vi "rqp_Msg_ToServer_6.vi"(4 "Show in Debugger?":bool=TRUE, 6 "Message Priority":T1=enum."Normal", 7 "Caller in":refnum<class "Worker.lvclass">, 8 "error in":errorcluster, 10 "Data in":T2, 11 "gRPC Client in":refnum<class "gRPC Client.lvclass">) -> (0 "error out":errorcluster, 3 "dup gRPC Client out":refnum<class "gRPC Client.lvclass">, 5 "dup Caller out":refnum<class "Worker.lvclass">)   [LabVIEW 2019, in "gRPC Client (template.proto).lvlib" / "gRPC Client.lvclass"]
doc: "This VI sends a <b>Public API Request</b> message to an MHL case of the Worker that owns this VI.\n---\nThis Request matches a gRPC message of the same name."
uses:
  gRPC Client.lvclass
  C:/Program Files (x86)/National Instruments/LabVIEW 2019/vi.lib/addons/_Workers/Library/Classes/Worker/Worker.lvclass
  <vilib>/addons/_Workers/Library/Classes/Worker/Worker.lvclass
  rqp_Msg_ToServer_6.ctl
  Generated_client/RPC Messages/w4lvgrpc_Msg_ToServer_6.ctl
  <vilib>/addons/_Workers/Library/Classes/Message/Priority.ctl
  <vilib>/addons/_Workers/Library/Case Label.ctl
  <vilib>/addons/_Workers/Library/Classes/Message Queue/Message Queue.lvclass
  <vilib>/addons/_Workers/Library/Workers.lvlib
  <vilib>/addons/_Workers/Library/Classes/Message/Message.lvclass
  Generated_client/Generated_client.lvlib
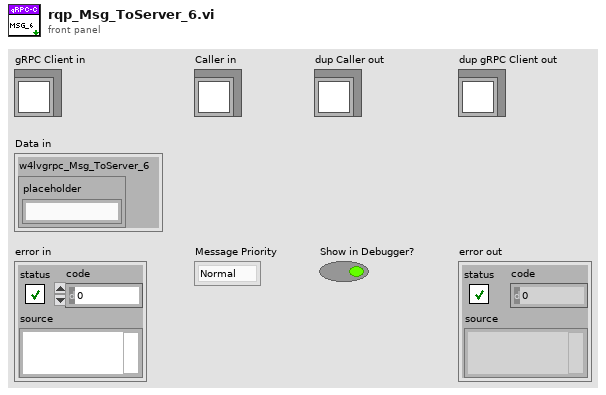
[diagram p1: front panel]
types:
  T1 = typedef "Workers.lvlib/Message.lvclass/Priority.ctl" = enum16{"Low", "Normal", "High"}
  T2 = typedef "gRPC Client (template.proto).lvlib/gRPC Client.lvclass/rqp_Msg_ToServer_6.ctl" = cluster{"w4lvgrpc_Msg_ToServer_6":T3}
  T3 = typedef "Generated_client.lvlib/w4lvgrpc_Msg_ToServer_6.ctl" = cluster{"placeholder":string}
  T4 = typedef "Workers.lvlib/Case Label.ctl" = string
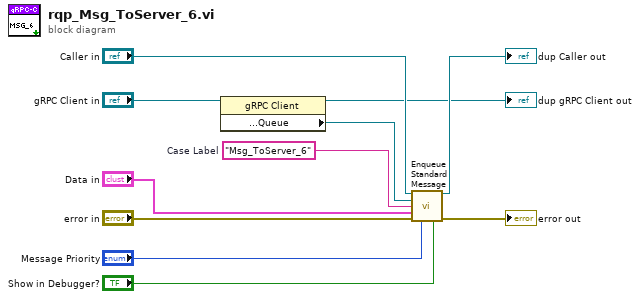
[diagram p0: block diagram]
diagram:
  w1 = T4 "Msg_ToServer_6"  # Case Label
  n1 = property class="gRPC Client"(reference="gRPC Client in") -> (reference out=→"dup gRPC Client out":refnum<class "gRPC Client.lvclass">, "Accessors:Read:Public API:Queue"=w2:refnum<class "Message Queue.lvclass">)  [unwired: 1 in, 1 out]
  n2 = call-dynamic "Enqueue Standard Message.vi"("Worker"="Caller in", "Message Queue"=w2, "Case Label"=w1, "Data"="Data in", "error in (no error)"="error in", "Priority (Normal)"="Message Priority", "Send Message to Debugger? (T)"="Show in Debugger?") -> ("dup Worker out"=→"dup Caller out":refnum<class "Worker.lvclass">, "error out"=→"error out":errorcluster)  [unwired: 7 in]
